vi "Enter String.vi"(8 "error in":errorcluster, 10 "Numeric Control":string, 11 "Message":string) -> (0 "error out":errorcluster, 2 "String Value":string)   [LabVIEW 2017]
panel:
  in  "OK Button":bool
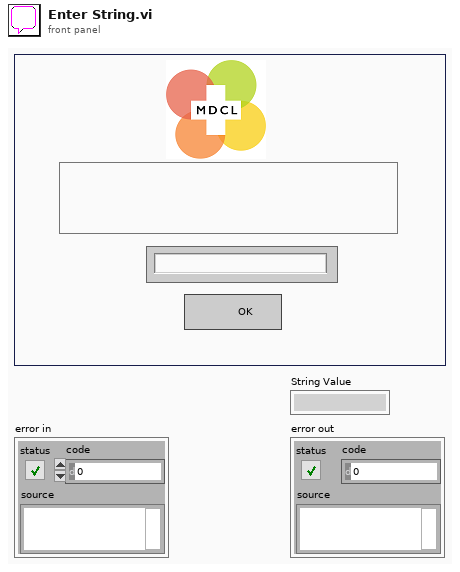
[diagram p1: front panel]
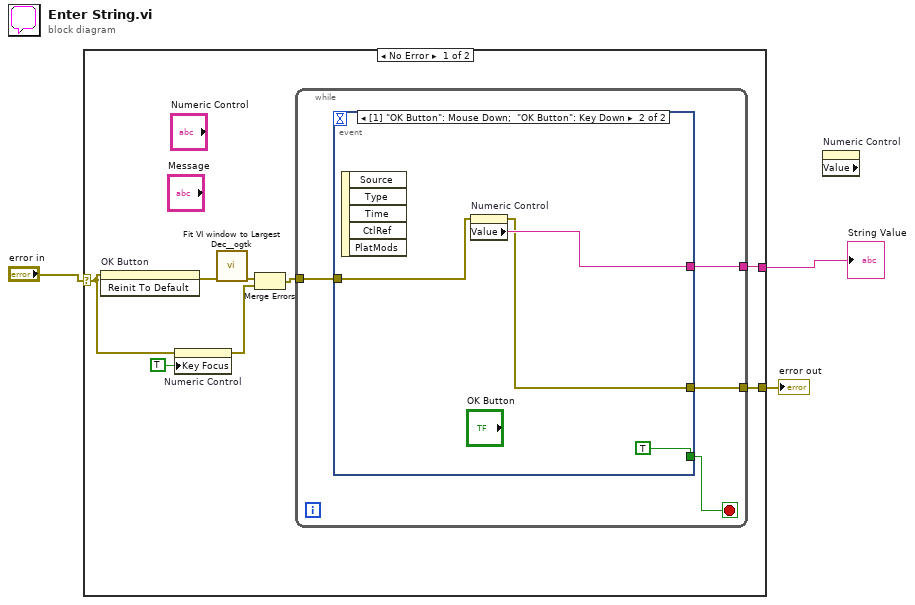
[diagram p0: block diagram]
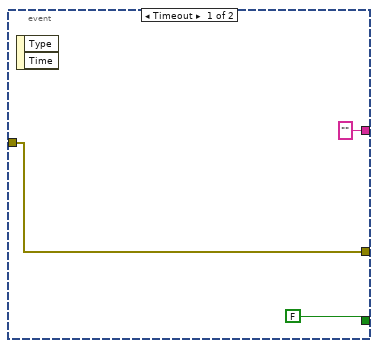
[diagram p2: hidden frame]
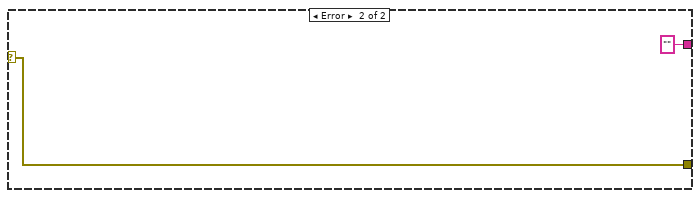
[diagram p3: hidden frame]
diagram:
  n1 = case shown="No Error" "error in" {
    selector: "error in" -> [w7 w24]
    tunnel: [w10 "" ("Value")] -> w3
    tunnel: [w9 w24] -> w1
    frame No Error {
      n2 = invoke on="OK Button" class="Bool (strict)" method="Reinit To Default"(error in=w7) -> (error out=w11:errorcluster)  [unwired: 2 in, 2 out]
      n3 = property on="Numeric Control" class="Str"(error in=w7, "Key Focus"=TRUE) -> (error out=w5:errorcluster)  [unwired: 1 in, 1 out]
      n4 = call <userlib>:"Fit VI window to Largest Dec__ogtk.vi"("error in (no error)"=w11) -> ("error out"=w6:errorcluster)  [unwired: 5 in, 1 out]
      n5 = Merge Errors(w6, w5) -> (w4:errorcluster)
      n6 = while {
        tunnel: w4 -> [w15]
        tunnel: [w14] -> w10
        tunnel: [w13] -> w9
        stop <- w12 stop-if-true
        n7 = event shown="[1] \"OK Button\": Mouse Down;  \"OK Button\": Key Down" {
          selector: _ -> [_ _]
          dyn-events: _ -> [_ _]
          timeout: _ -> [_ _]
          tunnel: w15 -> [w18 w20]
          tunnel: ["" ("Value") w21] -> w14
          tunnel: [w18 w19] -> w13
          tunnel: [FALSE TRUE] -> w12
          event Timeout {
            n8 = event-data() -> ()  [unwired: 1 in, 2 out]
          }
          event "OK Button": Mouse Down; "OK Button": Key Down {
            n9 = event-data() -> ()  [unwired: 1 in, 5 out]
            n10 = property on="Numeric Control" class="Str"(error in=w20) -> (error out=w19:errorcluster, "Value"=w21:string)  [unwired: 1 in, 1 out]
          }
        }
      }
    }
    frame Error {
    }
  }
  "String Value" <- w3
  "error out" <- w1
  n11 = property on="Numeric Control" class="Str" props=["Value"]() -> ()  [unwired: 2 in, 3 out]
